vi "GEvt-WatchdogThread.vi"(11 "WatchDogQ":refnum<queue>) -> ()   [LabVIEW 2020, in "Communicable State Machine.lvlib"]
uses:
  Communicable State Machine.lvlib
  GEvt-RequestDef.ctl
  _CSM_GlobalLog_MSG.ctl
  _CSM_Response Source Message.ctl
  _CSM_GlobalLog_MSG_TYPE.ctl
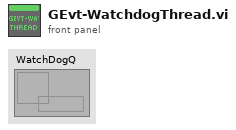
[diagram p1: front panel]
types:
  T1 = typedef "Communicable State Machine.lvlib/GEvt-RequestDef.ctl" = cluster{"Operation":enum16{"Obtain", "Destroy", "Force Destroy"}, "RespQ":refnum<queue>, "CSM Global Log Event":refnum<user-event>}
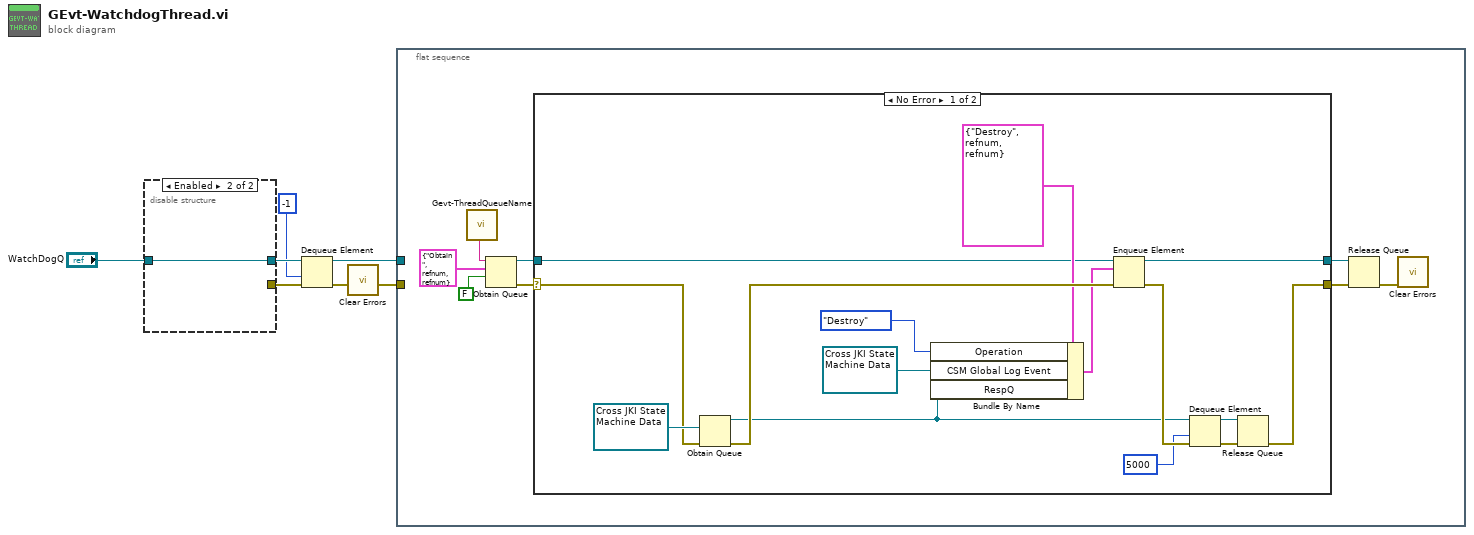
[diagram p0: block diagram]
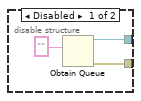
[diagram p3: hidden frame]
diagram:
  n1 = disable-structure shown="Enabled" {
    disable-tunnel: [w9 w11] -> w7
    disable-tunnel: [w8 _] -> w5
    disable-tunnel: "WatchDogQ" -> [_ w11]
    frame Disabled {
      n2 = Obtain Queue(element data type="") -> (queue out=w9:refnum<queue>, error out=w8:errorcluster)  [unwired: 4 in, 1 out]
    }
    frame Enabled {
    }
  }
  n3 = Dequeue Element(queue=w7, timeout in ms (-1)=-1, error in (no error)=w5) -> (queue out=w3:refnum<queue>, error out=w4:errorcluster)  [unwired: 2 out]
  n4 = call "Clear Errors.vi"("error in (no error)"=w4) -> ("error out"=w2:errorcluster)  [unwired: 5 in, 1 out]
  n5 = flat-sequence {
    tunnel: w2 -> [_]
    tunnel: w3 -> [_]
    frame #0 {
      n6 = call "Gevt-ThreadQueueName.vi"() -> ("ThreadQueueName"=w13:string)  [unwired: 5 in]
      n7 = Obtain Queue(name (unnamed)=w13, element data type=T1 {"Operation"=enum."Obtain", "RespQ"=refnum, "CSM Global Log Event"=refnum}, create if not found? (T)=FALSE) -> (queue out=w16:refnum<queue>, error out=w17:errorcluster)  [unwired: 2 in, 1 out]
      n8 = case shown="No Error" w17 {
        selector: w17 -> [w25 w35]
        tunnel: w16 -> [w26 w36]
        tunnel: [w24 w36] -> w15
        tunnel: [w23 w35] -> w14
        frame No Error {
          n9 = Obtain Queue(element data type=refnum<user-event> refnum ("CSM Global Log Event"), error in (no error)=w25) -> (queue out=w30:refnum<queue>, error out=w31:errorcluster)  [unwired: 3 in, 1 out]
          n10 = Bundle By Name(cluster=T1 {"Operation"=enum."Destroy", "RespQ"=refnum, "CSM Global Log Event"=refnum} ("element"), "Operation"=enum16{"Obtain", "Destroy", "Force Destroy"}."Destroy", "CSM Global Log Event"=refnum<user-event> refnum, "RespQ"=w30) -> (w28:T1)
          n11 = Enqueue Element(queue=w26, element=w28, error in (no error)=w31) -> (queue out=w24:refnum<queue>, error out=w32:errorcluster)  [unwired: 1 in, 1 out]
          n12 = Dequeue Element(queue=w30, timeout in ms (-1)=5000 ("timeout in ms (5000ms)"), error in (no error)=w32) -> (queue out=w34:refnum<queue>, error out=w33:errorcluster)  [unwired: 2 out]
          n13 = Release Queue(queue=w34, error in (no error)=w33) -> (error out=w23:errorcluster)  [unwired: 1 in, 2 out]
        }
        frame Error {
        }
      }
      n14 = Release Queue(queue=w15, error in (no error)=w14) -> (error out=w12:errorcluster)  [unwired: 1 in, 2 out]
      n15 = call "Clear Errors.vi"("error in (no error)"=w12) -> ()  [unwired: 5 in, 2 out]
    }
  }
